vi "Detect Brightness Maximum.vi"(5 "Bullseye Color":u32(colorbox)=16711808, 7 "Center Color":u32(colorbox)=9567230, 8 "error in (no error)":errorcluster, 9 "Threshold Max":sgl=255.0 min=0 max=255 step=1, 11 "Refnum In":T2) -> (0 "error out":errorcluster, 1 "Eccentricity vs. Threshold":cluster{i32[], dbl[]}(graph), 2 "Ellipses Out":T2, 3 "Bullseye Out":T2)   [LabVIEW 2017]
doc: "DETECT BRIGHTNESS MAXIMUM\nPrimary Author: Catherine Nicoloff (cnicolof@wellesley.edu)\n\nCore concept: Using the brightest spot in the field of view and a progression of thresholds, attempt to determine whether the camera is aligned with a flat field of view.\n\n-----\nDesign Philosophy: \n\nThis VI may require occasional configuration from the user for best performance.\n\nIf necessary, this SubVI can be opened during operation to display several tabs of debugging information as well as editable parameters.\n\nThis SubVI can also be run in stand-alone mode for testing by specifying a static image file to load from disk, provided no input image refnum is supplied.\n\n-----\nStructure:\n\n* Bright Spot Centering tab: Displays the image from the camera, overlaid with crosshairs indicating the image center and a bullseye indicating the center of the brightest region in the image. \n\nIf Refnum In is wired, the image displayed will be the input image. This will ordinarily be wired to accept a single frame from the camera.\n\nIf Refnum In is blank and File Path is valid, the VI will attempt to use the specified static image. This is useful for unit testing and debugging.\n\n * Bullseye Color: The color of the bullseye overlay. \n\n * Center Color: The color of the center crosshair overlay. \n\n* Progressive Threshold tab: Displays the results of a progressive series of thresholds applied to the original image.\n\n * Step Size: Set to 8 by default. Step the threshold from image mean to Threshold Max by the given interval.\n\n * Min. Objects: Set to 250 by default. The minimum number of objects necessary before attempting to fit an ellipse.\n\n * Threshold Max: Set to 255 by default. The maximum threshold value to step to. Use caution with this setting, as threshold values that are too high may create a false impression of misalignment.\n\n* Visualize Ellipses tab: Displays the camera image and the full set of detected objects for each threshold step.\n\n * Radius: Set to 8 by default. Radius of the overlay circles that mark the found objects.\n\n * Draw Mode: Set to Fill by default. Options are Fill or Frame. Whether to fill the overlay circles (default) or just draw the frame.\n\n * Object Display: Set to OFF (Fit) by default. Options are Fit or All. Draw just the objects used by the ellipse fit (Fit) or draw all the found objects (All).\n\n* Graphs tab: Displays three graphs to show the evolution of ellipse eccentricity and ellipse center coordinates with increasing threshold values."
uses:
  <vilib>/vision/Image Controls.llb/IMAQ Image.ctl
  <vilib>/vision/NI_Vision_Development_Module.lvlib
panel:
  out "Delta Y":dbl[](array[numeric])
  out "Delta X":dbl[](array[numeric])
  in  "Tab Control":T1(tab)
  out "Centering":T2(plugin-control)
  in  "File Path":path
  out "Find Objects":T2(plugin-control)
  in  "Step Size":i32=8
  in  "Min. Objects":i32=250
  out "e":sgl
  out "c":sgl
  out "b":sgl
  out "a":sgl
  out "Center X":dbl[](array[numeric])
  out "Center Y":dbl[](array[numeric])
  out "Eccentricity":dbl[](array[numeric])
  out "Threshold":i32[](array[numeric])
  out "Objects Found":i32[](array[numeric])
  in  "Object Display":bool
  out "Visualize Ellipses":T2(plugin-control)
  in  "Radius":i32=8
  in  "Draw Mode":u32(ring)=1 items=["Frame", "Fill"]
  out "Ellipse Center Y vs. Threshold":cluster{i32[], dbl[]}(graph)
  out "Ellipse Center X vs. Threshold":cluster{i32[], dbl[]}(graph)
  # "Author Credit:"
  # "Catherine Nicoloff (cnicolof@wellesley.edu)\n\nWellesley College\nAugust 2017"
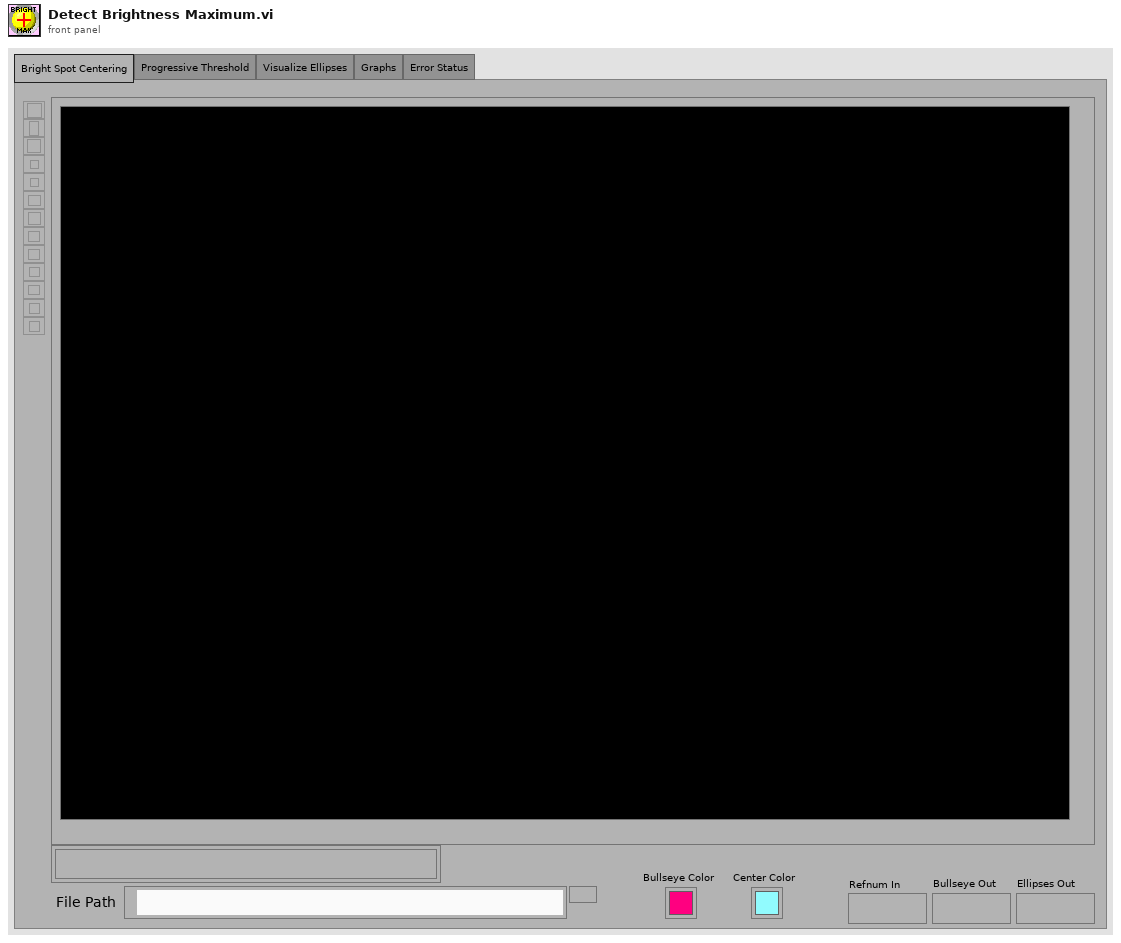
[diagram p1: front panel]
types:
  T1 = enum32{"Bright Spot Centering", "Progressive Threshold", "Visualize Ellipses", "Graphs", "Error Status"}
  T2 = typedef "IMAQ Image.ctl" = refnum<image>
  T3 = typedef "Image Type" = u32
  T4 = cluster{"histogram":u32[], "Minimal Value":sgl, "Maximal Value":sgl, "Starting Value":sgl, "Interval Width":sgl, "Mean Value":sgl, "Standard  Variation":sgl, "Area (pixels)":i32}
  T5 = cluster{"Objects":u16, "Threshold":i32, "Reject Border":bool, "Fill Holes":bool, "Min Object Size":bool, "Min Size":i32, "Max Object Size":bool, "Max Size":i32, "Show Search Area":bool, "Show Center":bool, "Show Bounding Box":bool}
  T6 = cluster{"Object Center":cluster{"X":sgl, "Y":sgl}, "Bounding Box":cluster{"X Left":i32, "Y Top":i32, "X Right":i32, "Y Bottom":i32}, "Area":sgl, "Orientation":sgl, "Aspect Ratio":sgl, "Nb Holes":i32}[]
  T7 = cluster{"Center":cluster{"X":sgl, "Y":sgl}, "Major Axis":cluster{"Point 1":cluster{"X":sgl, "Y":sgl}, "Point 2":cluster{"X":sgl, "Y":sgl}}, "Minor Axis":cluster{"Point 1":cluster{"X":sgl, "Y":sgl}, "Point 2":cluster{"X":sgl, "Y":sgl}}}
  T8 = cluster{"Point 1":cluster{"X":sgl, "Y":sgl}, "Point 2":cluster{"X":sgl, "Y":sgl}}
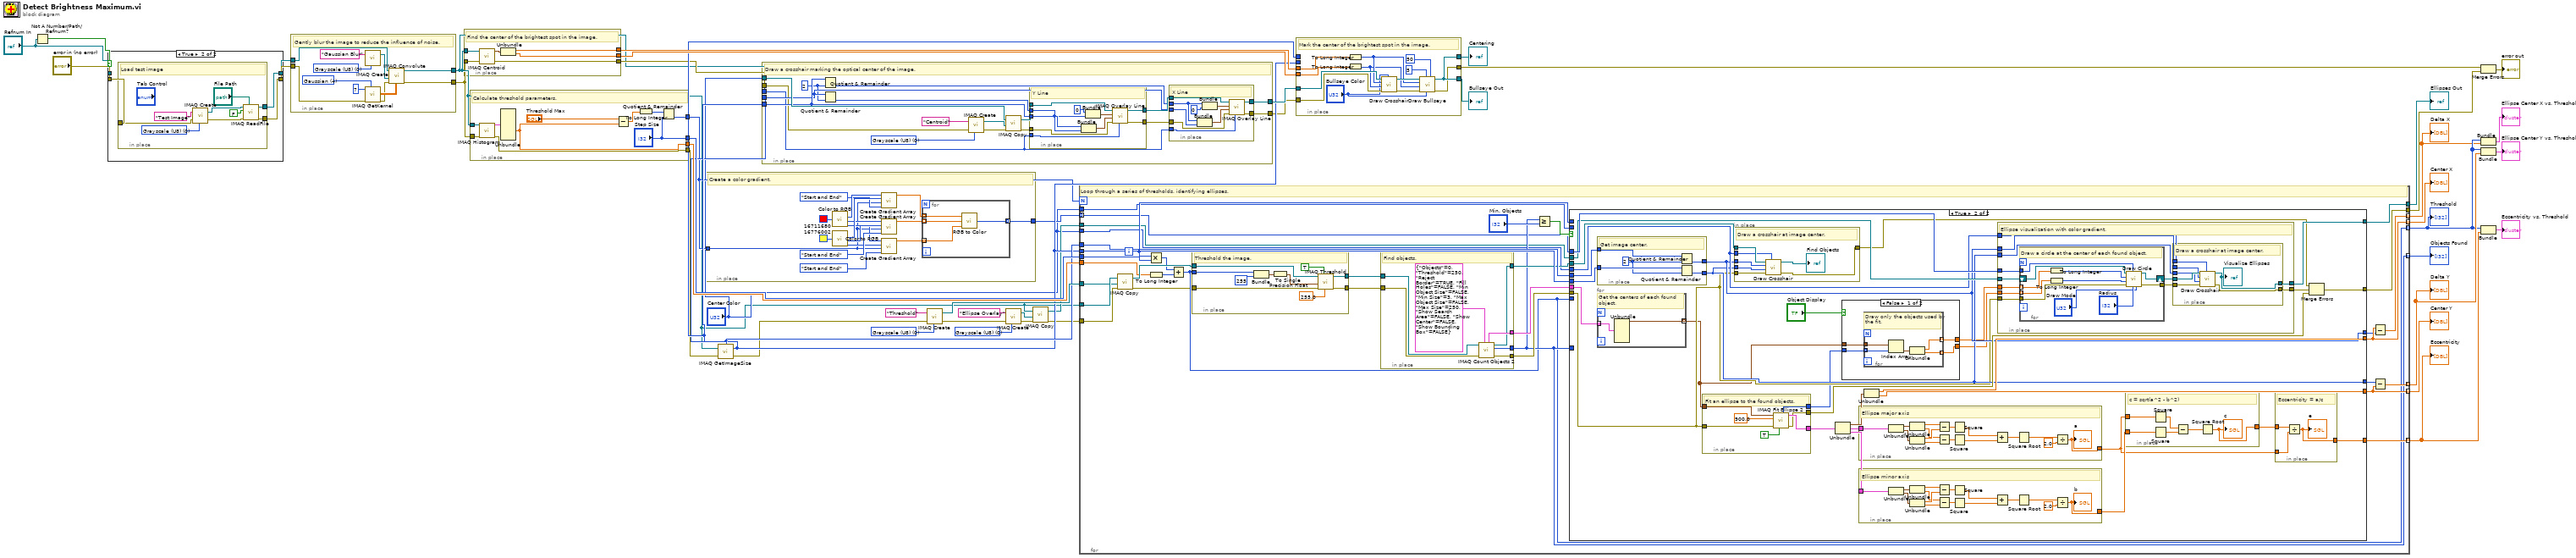
[diagram p0: block diagram]
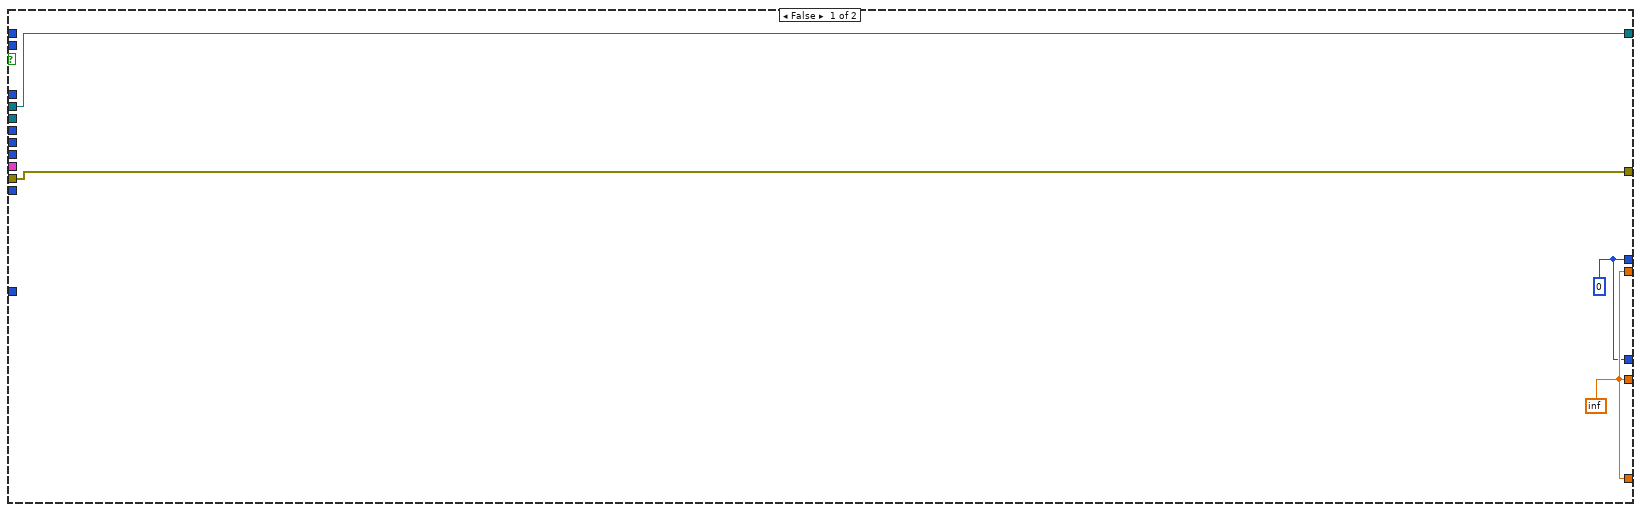
[diagram p2: hidden frame]
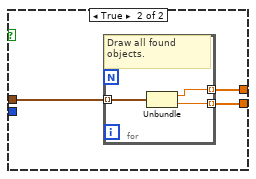
[diagram p3: hidden frame]
diagram:
  w20 = T3 0 items=["Grayscale (U8)", "Grayscale (I16)", "Grayscale (SGL)", "Complex (CSG)", "RGB (U32)", "HSL (U32)", "RGB (U64)", "Grayscale (U16)"] ("Image Type")
  w38 = T3 0 items=["Grayscale (U8)", "Grayscale (I16)", "Grayscale (SGL)", "Complex (CSG)", "RGB (U32)", "HSL (U32)", "RGB (U64)", "Grayscale (U16)"] ("Image Type")
  n1 = Not A Number/Path/Refnum?(number/path/refnum="Refnum In") -> (NaN/Path/Refnum?=w46:bool)
  n2 = case shown="True" w46 {
    tunnel: "error in (no error)" -> [w48 w52]
    tunnel: [w48 w50] -> w44
    tunnel: [w49 w51] -> w7
    tunnel: "Refnum In" -> [w49 _]
    frame False {
    }
    frame True {
      n3 = in-place {
        in-place-border: [w54] -> w51
        in-place-border: [w56] -> w50
        in-place-border: w52 -> [w55]
        w59 = T3 0 items=["Grayscale (U8)", "Grayscale (I16)", "Grayscale (SGL)", "Complex (CSG)", "RGB (U32)", "HSL (U32)", "RGB (U64)", "Grayscale (U16)"] ("Image Type")
        # "Load test image"
        n4 = call "IMAQ Create"("Image Name"="Test Image", "Image Type"=w59, "error in (no error)"=w55) -> ("New Image"=w60:T2, "error out"=w57:errorcluster)  [unwired: 2 in]
        n5 = call "IMAQ ReadFile"("File Path"="File Path", "error in (no error)"=w57, "Load Color Palette? (No)"=FALSE, "Image"=w60) -> ("error out"=w56:errorcluster, "Image Out"=w54:T2)  [unwired: 3 in, 3 out]
      }
    }
  }
  n6 = in-place {
    in-place-border: w44 -> [w70]
    in-place-border: w7 -> [w68]
    in-place-border: [w66] -> w6
    in-place-border: [w65] -> w5
    w64 = T3 0 items=["Grayscale (U8)", "Grayscale (I16)", "Grayscale (SGL)", "Complex (CSG)", "RGB (U32)", "HSL (U32)", "RGB (U64)", "Grayscale (U16)"] ("Image Type")
    w71 = u16 4 items=["Gradient"=1, "Laplacian"=2, "Smoothing"=3, "Gaussian"=4] ("Kernel Family")
    # "Gently blur the image to reduce the influence of noise."
    n7 = call "IMAQ Create"("Image Name"="Gaussian Blur", "Image Type"=w64) -> ("New Image"=w62:T2)  [unwired: 3 in, 1 out]
    n8 = call "IMAQ GetKernel"("Kernel Family"=w71, "error in (no error)"=w70, "Kernel Size (3,5,...)"=7) -> ("error out"=w67:errorcluster, "Kernel"=w69:sgl[][])  [unwired: 5 in, 2 out]
    n9 = call "IMAQ Convolute"("Kernel"=w69, "error in (no error)"=w67, "Image Dst"=w62, "Image Src"=w68) -> ("error out"=w65:errorcluster, "Image Dst Out"=w66:T2)  [unwired: 6 in]
  }
  n10 = in-place {
    in-place-border: w6 -> [w77]
    in-place-border: [w76] -> w43
    in-place-border: w5 -> [w75]
    in-place-border: [w73] -> w13
    in-place-border: [w74] -> w42
    # "Find the center of the brightest spot in the image."
    n11 = call "IMAQ Centroid"("error in (no error)"=w75, "Image"=w77) -> ("error out"=w73:errorcluster, "Centroid"=w78:cluster{"X Centroid":sgl, "Y Centroid":sgl})  [unwired: 2 in]
    n12 = Unbundle(w78) -> ("X Centroid"=w76:sgl, "Y Centroid"=w74:sgl)
  }
  n13 = in-place {
    in-place-border: [w86] -> w2
    in-place-border: ["Step Size"] -> w36
    in-place-border: w5 -> [w83]
    in-place-border: [w82] -> w30
    in-place-border: w6 -> [w81]
    in-place-border: [w80] -> w17
    # "Calculate threshold parameters."
    n14 = call "IMAQ Histogram"("error in (no error)"=w83, "Image"=w81) -> ("error out"=w86:errorcluster, "Histogram Report"=w88:T4)  [unwired: 8 in]
    n15 = Unbundle(w88) -> ("Mean Value"=w82:sgl)  [unwired: 7 out]
    n16 = Subtract(x="Threshold Max", y=w82) -> (x-y=w87:sgl)
    n17 = To Long Integer(number=w87) -> (32bit integer=w85:i32)
    n18 = Quotient & Remainder(x=w85, y="Step Size") -> (floor(x/y)=w80:i32)  [unwired: 1 out]
  }
  n19 = in-place {
    in-place-border: [w90] -> w16
    in-place-border: w17 -> [w89]
    # "Create a color gradient."
    n20 = call <vilib>:"Color to RGB.vi"("Color"=u32 16711680) -> ("R"=w103:u8, "G"=w99:u8, "B"=w95:u8)  [unwired: 1 out]
    n21 = call <vilib>:"Color to RGB.vi"("Color"=u32 16776002) -> ("R"=w104:u8, "G"=w100:u8, "B"=w96:u8)  [unwired: 1 out]
    n22 = call "Create Gradient Array.vi"("Values to Include"=enum16{"Start", "End", "Start and End", "None"}."Start and End", "Array Length"=w89, "End Value"=w104, "Start Value"=w103) -> ("Output Array"=w101:dbl[])  [unwired: 7 in]
    n23 = call "Create Gradient Array.vi"("Values to Include"=enum16{"Start", "End", "Start and End", "None"}."Start and End", "Array Length"=w89, "End Value"=w100, "Start Value"=w99) -> ("Output Array"=w97:dbl[])  [unwired: 7 in]
    n24 = call "Create Gradient Array.vi"("Values to Include"=enum16{"Start", "End", "Start and End", "None"}."Start and End", "Array Length"=w89, "End Value"=w96, "Start Value"=w95) -> ("Output Array"=w93:dbl[])  [unwired: 7 in]
    n25 = for {
      tunnel: w101 -> [w105] mode=indexing
      tunnel: w97 -> [w107] mode=indexing
      tunnel: w93 -> [w106] mode=indexing
      tunnel: [w108] -> w90 mode=indexing
      n26 = call <vilib>:"RGB to Color.vi"("B"=w106, "G"=w107, "R"=w105) -> ("Color"=w108:u32)
    }
  }
  n27 = call "IMAQ GetImageSize"("Image"=w6, "error in (no error)"=w2) -> ("Y Resolution"=w27:i32, "X Resolution"=w28:i32, "error out"=w1:errorcluster)  [unwired: 2 in]
  n28 = in-place {
    in-place-border: w28 -> [w116]
    in-place-border: w27 -> [w115]
    in-place-border: w6 -> [w118]
    in-place-border: [w125] -> w41
    in-place-border: [w123] -> w12
    in-place-border: w13 -> [w110]
    in-place-border: "Center Color" -> [w109]
    w121 = T3 0 items=["Grayscale (U8)", "Grayscale (I16)", "Grayscale (SGL)", "Complex (CSG)", "RGB (U32)", "HSL (U32)", "RGB (U64)", "Grayscale (U16)"] ("Image Type")
    w114 = 2
    # "Draw a crosshair marking the optical center of the image."
    n29 = Quotient & Remainder(x=w116, y=w114) -> (floor(x/y)=w113:i32)  [unwired: 1 out]
    n30 = Quotient & Remainder(x=w115, y=w114) -> (floor(x/y)=w112:i32)  [unwired: 1 out]
    n31 = call "IMAQ Create"("Image Name"="Centroid", "Image Type"=w121, "error in (no error)"=w110) -> ("New Image"=w122:T2, "error out"=w111:errorcluster)  [unwired: 2 in]
    n32 = call "IMAQ Copy"("error in (no error)"=w111, "Image Dst"=w122, "Image Src"=w118) -> ("error out"=w119:errorcluster, "Image Dst Out"=w117:T2)  [unwired: 3 in]
    n33 = in-place {
      in-place-border: [w133] -> w126
      in-place-border: [w132] -> w124
      in-place-border: w119 -> [w131]
      in-place-border: w117 -> [w130]
      in-place-border: w116 -> [w129]
      in-place-border: w112 -> [w128]
      in-place-border: w109 -> [w127]
      # "Y Line"
      n34 = Bundle("X Resolution"=w129, w128) -> (w134:cluster{"X Resolution":i32, i32})  [unwired: 1 in]
      n35 = Bundle(0, w128) -> (w135:cluster{i32, i32})  [unwired: 1 in]
      n36 = call "IMAQ Overlay Line"("Color"=w127, "error in (no error)"=w131, "End Point"=w134, "Start Point"=w135, "Image"=w130) -> ("error out"=w132:errorcluster, "Image Out"=w133:T2)  [unwired: 5 in]
    }
    n37 = in-place {
      in-place-border: w126 -> [w145]
      in-place-border: [w142] -> w125
      in-place-border: w124 -> [w141]
      in-place-border: [w140] -> w123
      in-place-border: w113 -> [w139]
      in-place-border: w115 -> [w138]
      in-place-border: w109 -> [w137]
      # "X Line"
      n38 = Bundle(w139, "Y Resolution"=w138) -> (w143:cluster{i32, "Y Resolution":i32})  [unwired: 1 in]
      n39 = Bundle(w139, 0) -> (w144:cluster{i32, i32})  [unwired: 1 in]
      n40 = call "IMAQ Overlay Line"("Color"=w137, "error in (no error)"=w141, "End Point"=w143, "Start Point"=w144, "Image"=w145) -> ("error out"=w140:errorcluster, "Image Out"=w142:T2)  [unwired: 5 in]
    }
  }
  n41 = call "IMAQ Create"("Image Name"="Threshold", "Image Type"=w38, "error in (no error)"=w1) -> ("New Image"=w37:T2, "error out"=w4:errorcluster)  [unwired: 2 in]
  n42 = call "IMAQ Create"("Image Name"="Ellipse Overlay", "Image Type"=w20, "error in (no error)"=w4) -> ("New Image"=w19:T2, "error out"=w18:errorcluster)  [unwired: 2 in]
  n43 = call "IMAQ Copy"("error in (no error)"=w18, "Image Dst"=w19, "Image Src"=w6) -> ("error out"=w3:errorcluster, "Image Dst Out"=w15:T2)  [unwired: 3 in]
  n44 = for {
    N: w17 -> [_]
    tunnel: w30 -> [w169]
    tunnel: [w161] -> w34 mode=indexing
    tunnel: [w157] -> w33 mode=indexing
    tunnel: [w177] -> w32 mode=indexing
    tunnel: w6 -> [w174]
    tunnel: w3 -> [w148]
    tunnel: w37 -> [w173]
    tunnel: w36 -> [w171]
    tunnel: [w166] -> w35
    tunnel: w28 -> [w165]
    tunnel: w27 -> [w164]
    tunnel: [w154] -> w24 mode=indexing
    tunnel: [w155] -> w29 mode=indexing
    tunnel: [w162] -> w23 mode=indexing
    tunnel: [w159] -> w26 mode=indexing
    tunnel: w16 -> [w153] mode=indexing
    tunnel: w15 -> [w152]
    tunnel: [w151] -> w14
    tunnel: "Center Color" -> [w150]
    tunnel: "Center Color" -> [w149]
    i -> [w156]
    # "Loop through a series of thresholds, identifying ellipses."
    n45 = call "IMAQ Copy"("error in (no error)"=w148, "Image Dst"=w173, "Image Src"=w174) -> ("error out"=w147:errorcluster, "Image Dst Out"=w172:T2)  [unwired: 3 in]
    n46 = Multiply(x=w156, y=w171) -> (x*y=w170:i32)
    n47 = To Long Integer(number=w169) -> (32bit integer=w168:i32)
    n48 = Add(x=w170, y=w168) -> (x+y=w154:i32)
    n49 = in-place {
      in-place-border: [w195] -> w176
      in-place-border: w147 -> [w194]
      in-place-border: [w193] -> w175
      in-place-border: w172 -> [w192]
      in-place-border: w154 -> [w191]
      # "Threshold the image."
      n50 = Bundle(w191, 255) -> (w190:cluster{i32, i32})  [unwired: 1 in]
      n51 = To Single Precision Float(number=w190) -> (single precision float=w189:cluster{sgl, sgl})
      n52 = call "IMAQ Threshold"("Replace Value"=sgl 255.0, "Keep/Replace Value (Replace)"=TRUE, "error in (no error)"=w194, "Range"=w189, "Image Src"=w192) -> ("error out"=w193:errorcluster, "Image Dst Out"=w195:T2)  [unwired: 5 in]
    }
    n53 = in-place {
      in-place-border: [w187] -> w167
      in-place-border: [w186] -> w180
      in-place-border: w176 -> [w185]
      in-place-border: w175 -> [w183]
      in-place-border: [w182] -> w155
      in-place-border: [w181] -> w163
      # "Find objects."
      n54 = call "IMAQ Count Objects 2"("Settings"=T5 {"Objects"=0, "Threshold"=250, "Reject Border"=TRUE, "Fill Holes"=FALSE, "Min Object Size"=FALSE, "Min Size"=3, "Max Object Size"=FALSE, "Max Size"=250, "Show Search Area"=FALSE, "Show Center"=FALSE, "Show Bounding Box"=FALSE}, "error in (no error)"=w183, "Image"=w185) -> ("error out"=w186:errorcluster, "Number of Objects"=w182:i32, "Image Out"=w181:T2, "Objects"=w187:T6)  [unwired: 4 in, 1 out]
    }
    n55 = Greater Or Equal?(x=w155, y="Min. Objects") -> (x >= y?=w178:bool)
    n56 = case shown="True" w178 {
      tunnel: w180 -> [w200 w210]
      tunnel: [w201 w224] -> w161
      tunnel: [w201 w223] -> w157
      tunnel: [w201 w225] -> w177
      tunnel: w167 -> [_ w221]
      tunnel: [w200 w217] -> w166
      tunnel: w165 -> [_ w216]
      tunnel: w164 -> [_ w215]
      tunnel: w163 -> [_ w209]
      tunnel: [w199 w212] -> w160
      tunnel: [w199 w211] -> w158
      tunnel: w156 -> [_ _]
      tunnel: w155 -> [_ _]
      tunnel: w154 -> [_ _]
      tunnel: w153 -> [_ w220]
      tunnel: w152 -> [w198 w219]
      tunnel: [w198 w213] -> w151
      tunnel: w150 -> [_ _]
      tunnel: w149 -> [_ w214]
      frame False {
        w199 = 0
        w201 = inf
      }
      frame True {
        n57 = in-place {
          in-place-border: w216 -> [w281]
          in-place-border: w215 -> [w280]
          in-place-border: [w278] -> w212
          in-place-border: [w277] -> w211
          w279 = 2
          # "Get image center."
          n58 = Quotient & Remainder(x=w281, y=w279) -> (floor(x/y)=w278:i32)  [unwired: 1 out]
          n59 = Quotient & Remainder(x=w280, y=w279) -> (floor(x/y)=w277:i32)  [unwired: 1 out]
        }
        n60 = for {
          tunnel: w221 -> [w290] mode=indexing
          tunnel: [w289] -> w205 mode=indexing
          # "Get the centers of each found object."
          n61 = Unbundle(w290) -> ("Object Center"=w289:cluster{"X":sgl, "Y":sgl})  [unwired: 5 out]
        }
        n62 = in-place {
          in-place-border: w210 -> [w295]
          in-place-border: [w294] -> w226
          in-place-border: [w293] -> w218
          in-place-border: w205 -> [w292]
          in-place-border: [w291] -> w204
          # "Fit an ellipse to the found objects."
          n63 = call "IMAQ Fit Ellipse 2"("Reject Outliers (FALSE)"=TRUE, "error in (no error)"=w295, "Minimum Score"=900.0, "Radial Points"=w292) -> ("error out"=w293:errorcluster, "Ellipse"=w294:T7, "Indexes of Points Used"=w291:i32[])  [unwired: 2 in, 3 out]
        }
        n64 = in-place {
          in-place-border: w209 -> [w288]
          in-place-border: [w286] -> w207
          in-place-border: w210 -> [w285]
          in-place-border: w214 -> [w284]
          in-place-border: w212 -> [w283]
          in-place-border: w211 -> [w282]
          # "Draw a crosshair at image center."
          n65 = call "Draw Crosshair.vi"("Color"=w284, "error in (no error)"=w285, "Y"=w282, "X"=w283, "Refnum in"=w288) -> ("error out"=w286:errorcluster, "Refnum out"=→"Find Objects":T2)  [unwired: 5 in]
        }
        n66 = Unbundle(w226) -> ("Center"=w231:cluster{"X":sgl, "Y":sgl}, "Major Axis"=w222:T8, "Minor Axis"=w230:T8)
        n67 = case shown="False" "Object Display" {
          tunnel: w205 -> [w235 w243]
          tunnel: w204 -> [w234 _]
          tunnel: [w233 w242] -> w203
          tunnel: [w232 w241] -> w202
          frame False {
            n68 = for {
              tunnel: w235 -> [w238]
              tunnel: [w240] -> w233 mode=indexing
              tunnel: [w239] -> w232 mode=indexing
              tunnel: w234 -> [w237] mode=indexing
              # "Draw only the objects used by the fit."
              n69 = Index Array(array=w238, index=w237) -> (element=w236:cluster{"X":sgl, "Y":sgl})
              n70 = Unbundle(w236) -> ("X"=w240:sgl, "Y"=w239:sgl)
            }
          }
          frame True {
            n71 = for {
              tunnel: w243 -> [w246] mode=indexing
              tunnel: [w245] -> w242 mode=indexing
              tunnel: [w244] -> w241 mode=indexing
              # "Draw all found objects."
              n72 = Unbundle(w246) -> ("X"=w245:sgl, "Y"=w244:sgl)
            }
          }
        }
        n73 = in-place {
          in-place-border: w222 -> [w336]
          in-place-border: [w322] -> w227
          # "Ellipse major axis"
          n74 = Unbundle(w336) -> ("Point 1"=w335:cluster{"X":sgl, "Y":sgl}, "Point 2"=w334:cluster{"X":sgl, "Y":sgl})
          n75 = Unbundle(w335) -> ("X"=w333:sgl, "Y"=w331:sgl)
          n76 = Unbundle(w334) -> ("X"=w332:sgl, "Y"=w330:sgl)
          n77 = Subtract(x=w333, y=w332) -> (x-y=w329:sgl)
          n78 = Subtract(x=w331, y=w330) -> (x-y=w328:sgl)
          n79 = Square(x=w329) -> (x^2=w326:sgl)
          n80 = Square(x=w328) -> (x^2=w327:sgl)
          n81 = Add(x=w326, y=w327) -> (x+y=w325:sgl)
          n82 = Square Root(x=w325) -> (sqrt(x)=w324:sgl)
          n83 = Divide(x=w324, y=sgl 2.0) -> (x/y=w322:sgl)
          "a" <- w322
        }
        n84 = in-place {
          in-place-border: w230 -> [w310]
          in-place-border: [w307] -> w229
          # "Ellipse minor axis"
          n85 = Unbundle(w310) -> ("Point 1"=w321:cluster{"X":sgl, "Y":sgl}, "Point 2"=w320:cluster{"X":sgl, "Y":sgl})
          n86 = Unbundle(w321) -> ("X"=w319:sgl, "Y"=w317:sgl)
          n87 = Unbundle(w320) -> ("X"=w318:sgl, "Y"=w316:sgl)
          n88 = Subtract(x=w319, y=w318) -> (x-y=w315:sgl)
          n89 = Subtract(x=w317, y=w316) -> (x-y=w314:sgl)
          n90 = Square(x=w315) -> (x^2=w312:sgl)
          n91 = Square(x=w314) -> (x^2=w313:sgl)
          n92 = Add(x=w312, y=w313) -> (x+y=w311:sgl)
          n93 = Square Root(x=w311) -> (sqrt(x)=w309:sgl)
          n94 = Divide(x=w309, y=sgl 2.0) -> (x/y=w307:sgl)
          "b" <- w307
        }
        n95 = Unbundle(w231) -> ("X"=w224:sgl, "Y"=w223:sgl)
        n96 = in-place {
          in-place-border: w220 -> [w258]
          in-place-border: w219 -> [w257]
          in-place-border: w214 -> [w256]
          in-place-border: [w253] -> w213
          in-place-border: w212 -> [w252]
          in-place-border: w211 -> [w251]
          in-place-border: w210 -> [w250]
          in-place-border: [w249] -> w208
          in-place-border: w203 -> [w248]
          in-place-border: w202 -> [w247]
          # "Ellipse visualization with color gradient."
          n97 = for {
            shift-right: [w273] -> w255
            shift-left: w257 -> [w274]
            tunnel: w258 -> [w268]
            tunnel: w250 -> [w272]
            tunnel: [w271] -> w254
            tunnel: w248 -> [w267] mode=indexing
            tunnel: w247 -> [w266] mode=indexing
            # "Draw a circle at the center of each found object."
            n98 = To Long Integer(number=w267) -> (32bit integer=w276:i32)
            n99 = To Long Integer(number=w266) -> (32bit integer=w275:i32)
            n100 = call "Draw Circle.vi"("Drawing Mode"="Draw Mode", "Radius"="Radius", "Object Color"=w268, "error in (no error)"=w272, "Y"=w275, "X"=w276, "Refnum in"=w274) -> ("error out"=w271:errorcluster, "Refnum out"=w273:T2)  [unwired: 3 in]
          }
          n101 = in-place {
            in-place-border: w256 -> [w265]
            in-place-border: w255 -> [w264]
            in-place-border: w254 -> [w263]
            in-place-border: [w262] -> w249
            in-place-border: [w261] -> w253
            in-place-border: w252 -> [w260]
            in-place-border: w251 -> [w259]
            # "Draw a crosshair at image center."
            n102 = call "Draw Crosshair.vi"("Color"=w265, "error in (no error)"=w263, "Y"=w259, "X"=w260, "Refnum in"=w264) -> ("error out"=w262:errorcluster, "Refnum out"=w261:T2)  [unwired: 5 in]
            "Visualize Ellipses" <- w261
          }
        }
        n103 = in-place {
          in-place-border: w227 -> [w306]
          in-place-border: w229 -> [w305]
          in-place-border: [w301] -> w228
          # "c = sqrt(a^2 - b^2)"
          n104 = Square(x=w306) -> (x^2=w304:sgl)
          n105 = Square(x=w305) -> (x^2=w303:sgl)
          n106 = Subtract(x=w304, y=w303) -> (x-y=w302:sgl)
          n107 = Square Root(x=w302) -> (sqrt(x)=w301:sgl)
          "c" <- w301
        }
        n108 = in-place {
          in-place-border: w228 -> [w300]
          in-place-border: w227 -> [w299]
          in-place-border: [w298] -> w225
          # "Eccentricity = a/c"
          n109 = Divide(x=w300, y=w299) -> (x/y=w298:sgl)
          "e" <- w298
        }
        n110 = Merge Errors(w207, w208, w218) -> (w217:errorcluster)
      }
    }
    n111 = Subtract(x=w161, y=w160) -> (x-y=w162:dbl)
    n112 = Subtract(x=w158, y=w157) -> (x-y=w159:dbl)
  }
  "Center X" <- w34
  "Center Y" <- w33
  "Eccentricity" <- w32
  "Threshold" <- w24
  "Objects Found" <- w29
  "Delta X" <- w23
  "Delta Y" <- w26
  "Ellipses Out" <- w14
  n113 = in-place {
    in-place-border: w43 -> [w349]
    in-place-border: w42 -> [w348]
    in-place-border: w28 -> [_]
    in-place-border: w27 -> [_]
    in-place-border: w41 -> [w347]
    in-place-border: w12 -> [w345]
    in-place-border: [w343] -> w10
    in-place-border: [w343] -> w9
    in-place-border: [w342] -> w8
    # "Mark the center of the brightest spot in the image."
    n114 = To Long Integer(number=w349) -> (32bit integer=w341:i32)
    n115 = To Long Integer(number=w348) -> (32bit integer=w340:i32)
    n116 = call "Draw Crosshair.vi"("Color"="Bullseye Color", "error in (no error)"=w345, "Y"=w340, "X"=w341, "Refnum in"=w347) -> ("error out"=w344:errorcluster, "Refnum out"=w346:T2)  [unwired: 5 in]
    n117 = call "Draw Bullseye.vi"("Step Size"=50, "Bullseye Color"="Bullseye Color", "Number of Circles"=5, "error in (no error)"=w344, "Y"=w340, "X"=w341, "Refnum in"=w346) -> ("error out"=w342:errorcluster, "Refnum out"=w343:T2)  [unwired: 3 in]
  }
  "Bullseye Out" <- w9
  "Centering" <- w10
  n118 = Merge Errors(w8, w35) -> (→"error out":errorcluster)
  n119 = Bundle(w24, w23) -> (→"Ellipse Center X vs. Threshold":cluster{i32[], dbl[]})  [unwired: 1 in]
  n120 = Bundle(w24, w26) -> (→"Ellipse Center Y vs. Threshold":cluster{i32[], dbl[]})  [unwired: 1 in]
  n121 = Bundle(w24, w32) -> (→"Eccentricity vs. Threshold":cluster{i32[], dbl[]})  [unwired: 1 in]
